vi "Send Evaluate Save Test Executive.vi"(7 "Message Priority (Normal)":T2=enum."Normal", 8 "error in (no error)":errorcluster, 10 "Create Test Executive":T1, 11 "Message Enqueuer":refnum<class "Message Enqueuer.lvclass">) -> (0 "error out":errorcluster, 3 "Message Enqueuer out":refnum<class "Message Enqueuer.lvclass">)   [LabVIEW 2017, in "Evaluate Save Test Executive Msg.lvclass"]
doc: "This VI sends the message to an actor."
uses:
  <vilib>/gpm_packages/@cs/Test-executive-builder/Source/Test Executive Builder Model/Test Executive Builder Model Messages/Evaluate Save Test Executive Msg/Evaluate Save Test Executive Msg.lvclass
  <vilib>/ActorFramework/Message Enqueuer/Message Enqueuer.lvclass
  <vilib>/ActorFramework/Message Enqueuer/Message Priority.ctl
  <vilib>/gpm_packages/@cs/Test-executive-builder/Source/Application Dependencies/Create Test Executive.ctl
  C:/Program Files/National Instruments/LabVIEW 2017/vi.lib/ActorFramework/Message/Message.lvclass
  <vilib>/gpm_packages/@cs/Test-executive-builder/Source/Test Executive Builder Model/Test Executive Builder Model Messages/Evaluate Save Test Executive Msg/Evaluate Save Test Executive Msg.lvclass/Evaluate Save Test Executive Msg.ctl
  <vilib>/ActorFramework/Message Enqueuer/Message Enqueuer.lvclass/Message Enqueuer.ctl
  <vilib>/ActorFramework/Message Priority Queue/Priority Enqueue.vi
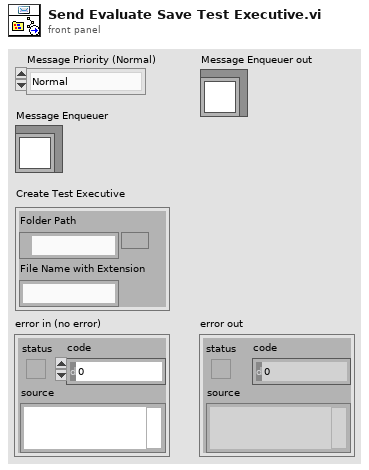
[diagram p1: front panel]
types:
  T1 = typedef "Create Test Executive.ctl" = cluster{"Folder Path":path, "File Name with Extension":string}
  T2 = typedef "Actor Framework.lvlib/Message Enqueuer.lvclass/Message Priority.ctl" = enum16{"Low", "Normal", "High"}
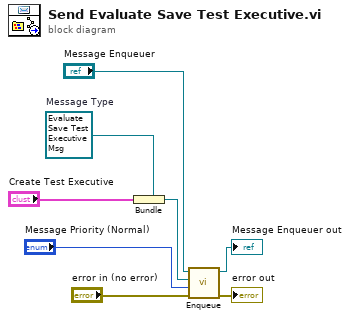
[diagram p0: block diagram]
diagram:
  w5 = refnum<class "Evaluate Save Test Executive Msg.lvclass"> refnum  # Message Type
  n1 = Bundle(cluster=w5, "Create Test Executive") -> (w4:refnum<class "Evaluate Save Test Executive Msg.lvclass">)
  n2 = call <vilib>:"Enqueue.vi"("error in (no error)"="error in (no error)", "Message Priority (Normal)"="Message Priority (Normal)", "Message"=w4, "Message Enqueuer in"="Message Enqueuer") -> ("error out"=→"error out":errorcluster, "Message Enqueuer out"=→"Message Enqueuer out":refnum<class "Message Enqueuer.lvclass">)  [unwired: 6 in]
